vi "Agilent 3446X Series Acquire Multiple.vi"() -> ()   [LabVIEW 2013]
doc: "This example shows how to configure a measurement and take multiple readings."
uses:
  <instrlib>/Agilent 3446X Series/Public/Data/Read (Multiple Points).vi
  <instrlib>/Agilent 3446X Series/Agilent 3446X Series.lvlib
panel:
  in  "Timeout (10000 ms)":i32=10000 format="%#.6g"
  in  "Sample Count (1)":i32=1
  in  "Measurement Function (10: Voltage DC)":i32(ring)=10 items=["Continuity", "Current AC", "Current DC", "Diode", "Frequency", "Resistance 4-wire", "Period", "Resistance 2-wire", "Temperature", "Voltage AC", "Voltage DC", "Voltage DC Ratio", "Capacitance"]
  in  "VISA resource name":refnum<visa-resource-name>
  out "Measurements":dbl[](array[numeric])
  # "(c) 2013-2021 National Instruments.  ALL RIGHTS RESERVED."
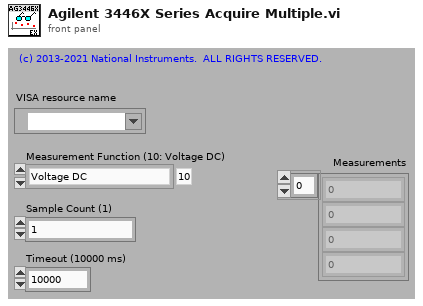
[diagram p1: front panel]
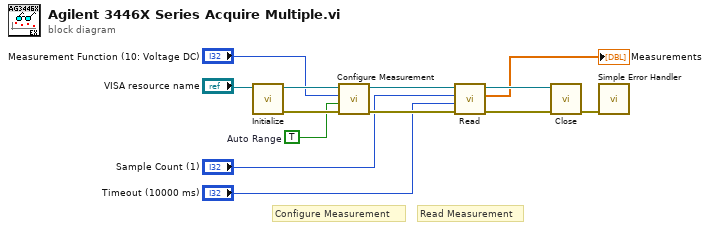
[diagram p0: block diagram]
diagram:
  w10 = TRUE  # Auto Range
  # "Read Measurement"
  # "Configure Measurement"
  n1 = call <instrlib>:"Initialize.vi"("VISA resource name"="VISA resource name") -> ("error out"=w11:errorcluster, "VISA resource name out"=w12:refnum<visa-resource-name>)  [unwired: 4 in, 5 out]
  n2 = call <instrlib>:"Configure Measurement.vi"("error in (no error)"=w11, "Auto Range (T: Enable)"=w10, "Measurement Function (10: Voltage DC)"="Measurement Function (10: Voltage DC)", "VISA resource name"=w12) -> ("error out"=w8:errorcluster, "VISA resource name out"=w7:refnum<visa-resource-name>)  [unwired: 2 in, 4 out]
  n3 = call-poly <instrlib>:"Read.vi"("error in (no error)"=w8, "Timeout (10000 ms)"="Timeout (10000 ms)", "Sample Count (1)"="Sample Count (1)", "VISA resource name"=w7) -> ("error out"=w9:errorcluster, "Measurements"=→"Measurements":dbl[], "VISA resource name out"=w6:refnum<visa-resource-name>)  [unwired: 5 out]
  n4 = call <instrlib>:"Close.vi"("error in (no error)"=w9, "VISA resource name"=w6) -> ("error out"=w13:errorcluster)  [unwired: 9 out]
  n5 = call <vilib>:"Simple Error Handler.vi"("error in (no error)"=w13) -> ()  [unwired: 1 in, 8 out]
